vi "test - Convert config array - SGL - 1.vi"(8 "error in (no error)":errorcluster, 11 "TestCase in":refnum<class "Create New Assert Tester.lvclass">) -> (0 "error out":errorcluster, 3 "TestCase out":refnum<class "Create New Assert Tester.lvclass">)   [LabVIEW 2016, in "Create New Assert Tester.lvclass"]
uses:
  Create New Assert Tester.lvclass
  Plugins/Utility/Assert Build Configuration.ctl
  Core/Assert API Components/Failure Actions.ctl
  <vilib>/Utility/Data Type/Type Definitions/Data Type.ctl
  Plugins/Utility/Assert Scripting Configuration.ctl
  <vilib>/addons/_JKI Toolkits/VI Tester/TestCase.llb/TestCase.lvclass
  <vilib>/Utility/Data Type/NI_Data Type.lvlib
  Core/Assert API Components/Assert API Components.lvlib
  C:/Program Files (x86)/National Instruments/LabVIEW 2016/vi.lib/addons/_JKI Toolkits/VI Tester/TestCase.llb/TestCase.lvclass
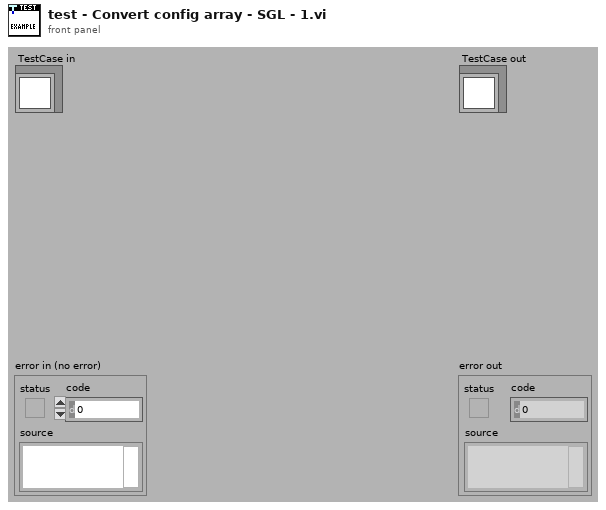
[diagram p1: front panel]
types:
  T1 = typedef "Assert Build Configuration.ctl" = cluster{"Assert Name":string, "Operation":string, "Comparison Value 1":string, "Comparison Value 2":string, "Comment":string, "Default Failure Action":T2, "Description":string, "Operation Display":string, "Active":bool, "Data Type":T3}
  T2 = typedef "Assert API Components.lvlib/Failure Actions.ctl" = enum16{"None", "Log To File", "Pause Execution", "Abort Execution"}
  T3 = typedef "NI_Data Type.lvlib/Data Type.ctl" = enum8{"Invalid Type", "Void", "I8", "I16", "I32", "I64", "U8", "U16", "U32", "U64", "Single Float", "Double Float", "Extended Float", "Single Complex", "Double Complex", "Extended Complex", "Enum U8", "Enum U16", "Enum U32", "Enum U64", "Single Float With Unit", "Double Float With Unit", "Extended Float With Unit", "Single Complex with Unit", "Double Complex with Unit", "Extended Complex with Unit", "Boolean", "String", "Path", "Picture", "Tag", "Array", "Cluster", "Variant", "LV Variant", "Waveform", "Timestamp", "Digital Waveform", "Digital Data", "ExpressData", "Refnum", "External Data", "VI", "Poly VI", "LabVIEW Class Instance", "Fixed Point"}
  T4 = enum16{"None", "Log To File", "Pause Execution", "Abort Execution"}
  T5 = typedef "Assert Scripting Configuration.ctl" = cluster{"Assert Name":string, "Comment":string, "Numeric Operation":string, "Type":T3, "String Operation":string, "DBL Comparison Value 1":dbl, "DBL Comparison Value 2":dbl, "I32 Comparison Value 1":i32, "I32 Comparison Value 2":i32, "Creator":string, "Creation Timestamp":timestamp, "String Comparison Value":string, "Description":string, "Default Failure Action":enum16{"None", "Log To File", "Pause Execution", "Abort Execution"}, "Boolean Comparison Value":bool, "I8 Comparison Value 1":i8, "I8 Comparison Value 2":i8, "I16 Comparison Value 1":i16, "I16 Comparison Value 2":i16, "I64 Comparison Value 1":i64, "I64 Comparison Value 2":i64, "U8 Comparison Value 1":u8, "U8 Comparison Value 2":u8, "U16 Comparison Value 1":u16, "U16 Comparison Value 2":u16, "U32 Comparison Value 1":u32, "U32 Comparison Value 2":u32, "U64 Comparison Value 1":u64, "U64 Comparison Value 2":u64, "EXT Comparison Value 1":ext, "EXT Comparison Value 2":ext, "SGL Comparison Value 1":sgl, "SGL Comparison Value 2":sgl}
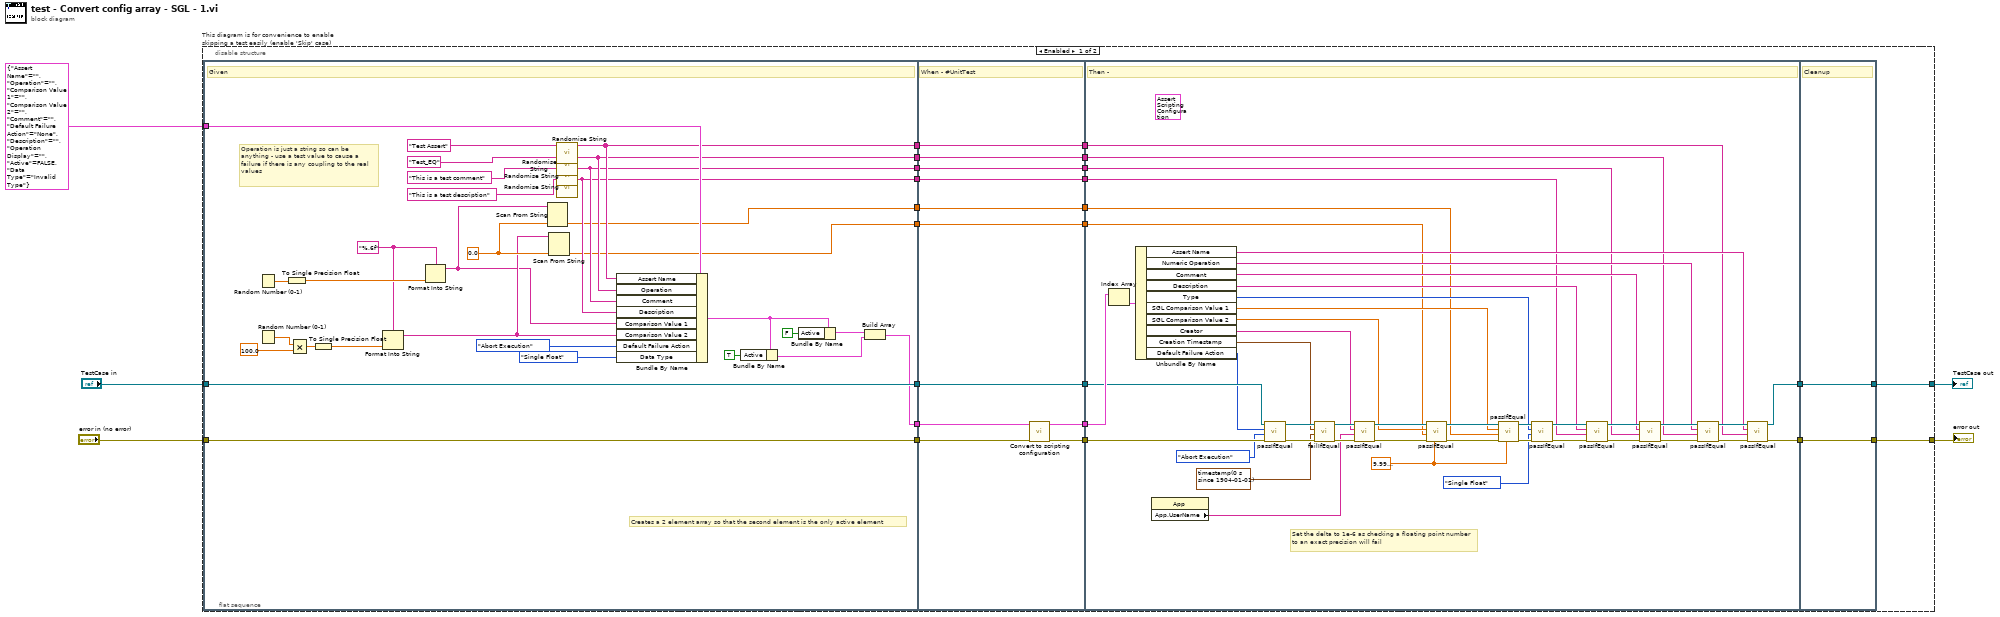
[diagram p0: block diagram]
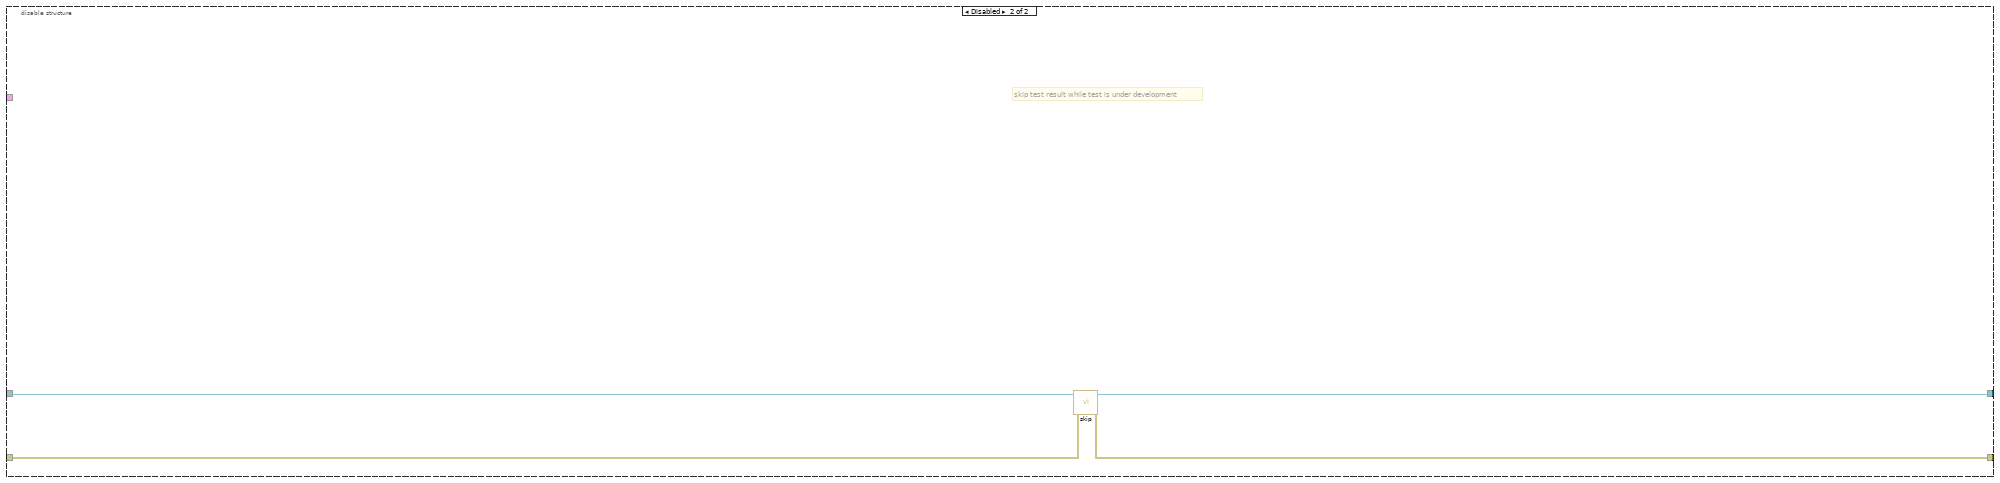
[diagram p2: hidden frame]
diagram:
  n1 = disable-structure "This diagram is for convenience to enable skipping a test easily (enable 'Skip' case)" shown="Enabled" {
    disable-tunnel: "TestCase in" -> [w24 w123]
    disable-tunnel: [w21 w121] -> w2
    disable-tunnel: [w22 w122] -> w4
    disable-tunnel: "error in (no error)" -> [w23 w120]
    disable-tunnel: T1 {"Assert Name"="", "Operation"="", "Comparison Value 1"="", "Comparison Value 2"="", "Comment"="", "Default Failure Action"=enum."None", "Description"="", "Operation Display"="", "Active"=FALSE, "Data Type"=enum."Invalid Type"} ("Assert Build Configuration") -> [w19 _]
    frame Enabled {
      n2 = flat-sequence {
        tunnel: w23 -> [w60]
        tunnel: w24 -> [w61]
        tunnel: [w61] -> w30
        tunnel: [w60] -> w29
        tunnel: w19 -> [w59]
        tunnel: [w54] -> w18
        tunnel: [w46] -> w16
        tunnel: [w45] -> w14
        tunnel: [w44] -> w12
        tunnel: [w43] -> w10
        tunnel: [w32] -> w8
        tunnel: [w31] -> w6
        tunnel: [w72] -> w28
        tunnel: [w70] -> w27
        tunnel: w30 -> [w72]
        tunnel: w29 -> [w71]
        tunnel: [w69] -> w20
        tunnel: w18 -> [w68]
        tunnel: [w67] -> w17
        tunnel: w16 -> [w67]
        tunnel: [w66] -> w15
        tunnel: w14 -> [w66]
        tunnel: [w65] -> w13
        tunnel: w12 -> [w65]
        tunnel: [w64] -> w11
        tunnel: w10 -> [w64]
        tunnel: [w63] -> w9
        tunnel: w8 -> [w63]
        tunnel: [w62] -> w7
        tunnel: w6 -> [w62]
        tunnel: [w81] -> w26
        tunnel: [w83] -> w25
        tunnel: w28 -> [w112]
        tunnel: w27 -> [w117]
        tunnel: w20 -> [w115]
        tunnel: w17 -> [w76]
        tunnel: w15 -> [w77]
        tunnel: w13 -> [w78]
        tunnel: w11 -> [w79]
        tunnel: w9 -> [w74]
        tunnel: w7 -> [w75]
        tunnel: [w118] -> w22
        tunnel: [w119] -> w21
        tunnel: w26 -> [w119]
        tunnel: w25 -> [w118]
        frame #0 {
          w35 = sgl 0.0 ("double precision float")
          w36 = "%.6f" ("format string")
          # "Creates a 2 element array so that the second element is the only active element"
          # "Operation is just a string so can be anything - use a test value to cause a failure if there is any coupling to the real values"
          # "Given"
          n3 = Random Number (0-1)() -> (number: 0 to 1=w42:dbl)
          n4 = Random Number (0-1)() -> (number: 0 to 1=w41:dbl)
          n5 = To Single Precision Float(number=w42) -> (single precision float=w37:sgl)
          n6 = Multiply(x=w41, y=100.0) -> (x*y=w39:dbl)
          n7 = To Single Precision Float(number=w39) -> (single precision float=w38:sgl)
          n8 = Format Into String(format string=w36, w38) -> (resulting string=w34:string)  [unwired: 2 in, 1 out]
          n9 = Format Into String(format string=w36, w37) -> (resulting string=w33:string)  [unwired: 2 in, 1 out]
          n10 = Scan From String(input string=w33, default 1=w35) -> (output 1=w32:sgl)  [unwired: 3 in, 3 out]
          n11 = Scan From String(input string=w34, default 1=w35) -> (output 1=w31:sgl)  [unwired: 3 in, 3 out]
          n12 = call "Randomise String.vi"("String in"="Test Assert" ("Assert Name")) -> ("String out"=w46:string)  [unwired: 10 in]
          n13 = call "Randomise String.vi"("String in"="Test_EQ" ("Operation")) -> ("String out"=w45:string)  [unwired: 10 in]
          n14 = call "Randomise String.vi"("String in"="This is a test comment" ("Comment")) -> ("String out"=w44:string)  [unwired: 10 in]
          n15 = call "Randomise String.vi"("String in"="This is a test description" ("Comment")) -> ("String out"=w43:string)  [unwired: 10 in]
          n16 = Bundle By Name(cluster=w59, "Assert Name"=w46, "Operation"=w45, "Comment"=w44, "Description"=w43, "Comparison Value 1"=w33, "Comparison Value 2"=w34, "Default Failure Action"=Failure_Actions."Abort Execution", "Data Type"=Data_Type."Single Float") -> (w51:T1)
          n17 = Bundle By Name(cluster=w51, "Active"=TRUE) -> (w49:T1)
          n18 = Bundle By Name(cluster=w51, "Active"=FALSE) -> (w53:T1)
          n19 = Build Array(w53, w49) -> (w54:T1[])
        }
        frame #1 {
          # "When - #UnitTest"
          n20 = call "Convert to scripting configuration.vi"("error in (no error)"=w71, "Multiple Assert Configuration"=w68) -> ("error out"=w70:errorcluster, "Array"=w69:T5[])  [unwired: 7 in, 1 out]
        }
        frame #2 {
          w73 = sgl 1e-06
          (unwired) T5 {"Assert Name"="", "Comment"="", "Numeric Operation"="", "Type"=enum."Invalid Type", "String Operation"="", "DBL Comparison Value 1"=0.0, "DBL Comparison Value 2"=0.0, "I32 Comparison Value 1"=0, "I32 Comparison Value 2"=0, "Creator"="", "Creation Timestamp"=timestamp(0 s since 1904-01-01), "String Comparison Value"="", "Description"="", "Default Failure Action"=enum."None", "Boolean Comparison Value"=FALSE, "I8 Comparison Value 1"=0, "I8 Comparison Value 2"=0, "I16 Comparison Value 1"=0, "I16 Comparison Value 2"=0, "I64 Comparison Value 1"=0, "I64 Comparison Value 2"=0, "U8 Comparison Value 1"=0, "U8 Comparison Value 2"=0, "U16 Comparison Value 1"=0, "U16 Comparison Value 2"=0, "U32 Comparison Value 1"=0, "U32 Comparison Value 2"=0, "U64 Comparison Value 1"=0, "U64 Comparison Value 2"=0, "EXT Comparison Value 1"=0.0, "EXT Comparison Value 2"=0.0, "SGL Comparison Value 1"=0.0, "SGL Comparison Value 2"=0.0} ("Assert Scripting Configuration")
          # "Set the delta to 1e-6 as checking a floating point number to an exact precision will fail"
          # "Then -"
          n21 = Index Array(array=w115) -> (element=w114:T5)  [unwired: 1 in]
          n22 = Unbundle By Name(w114) -> ("Assert Name"=w80:string, "Numeric Operation"=w89:string, "Comment"=w90:string, "Description"=w91:string, "Type"=w92:T3, "SGL Comparison Value 1"=w99:sgl, "SGL Comparison Value 2"=w100:sgl, "Creator"=w101:string, "Creation Timestamp"=w87:timestamp, "Default Failure Action"=w110:T4)
          n23 = property class="App"() -> ("App.UserName"=w85:string)  [unwired: 2 in, 2 out]
          n24 = call-dynamic "passIfEqual.vi"("error in (no error)"=w117, "y"=T4."Abort Execution" ("Default Failure Action"), "x"=w110, "TestCase in"=w112) -> ("error out"=w113:errorcluster, "TestCase out"=w111:refnum<class "Create New Assert Tester.lvclass">)  [unwired: 6 in]
          n25 = call-dynamic "failIfEqual.vi"("error in (no error)"=w113, "y"=timestamp(0 s since 1904-01-01) ("Creation Timestamp"), "x"=w87, "TestCase in"=w111) -> ("error out"=w116:errorcluster, "TestCase out"=w106:refnum<class "Create New Assert Tester.lvclass">)  [unwired: 6 in]
          n26 = call-dynamic "passIfEqual.vi"("error in (no error)"=w116, "y"=w85, "x"=w101, "TestCase in"=w106) -> ("error out"=w107:errorcluster, "TestCase out"=w105:refnum<class "Create New Assert Tester.lvclass">)  [unwired: 6 in]
          n27 = call-dynamic "passIfEqual.vi"("delta (optional)"=w73, "error in (no error)"=w107, "y"=w75, "x"=w100, "TestCase in"=w105) -> ("error out"=w108:errorcluster, "TestCase out"=w103:refnum<class "Create New Assert Tester.lvclass">)  [unwired: 5 in]
          n28 = call-dynamic "passIfEqual.vi"("delta (optional)"=w73, "error in (no error)"=w108, "y"=w74, "x"=w99, "TestCase in"=w103) -> ("error out"=w104:errorcluster, "TestCase out"=w97:refnum<class "Create New Assert Tester.lvclass">)  [unwired: 5 in]
          n29 = call-dynamic "passIfEqual.vi"("error in (no error)"=w104, "y"=Data_Type."Single Float" ("Data Type"), "x"=w92, "TestCase in"=w97) -> ("error out"=w98:errorcluster, "TestCase out"=w96:refnum<class "Create New Assert Tester.lvclass">)  [unwired: 6 in]
          n30 = call-dynamic "passIfEqual.vi"("error in (no error)"=w98, "y"=w79, "x"=w91, "TestCase in"=w96) -> ("error out"=w102:errorcluster, "TestCase out"=w94:refnum<class "Create New Assert Tester.lvclass">)  [unwired: 6 in]
          n31 = call-dynamic "passIfEqual.vi"("error in (no error)"=w102, "y"=w78, "x"=w90, "TestCase in"=w94) -> ("error out"=w95:errorcluster, "TestCase out"=w93:refnum<class "Create New Assert Tester.lvclass">)  [unwired: 6 in]
          n32 = call-dynamic "passIfEqual.vi"("error in (no error)"=w95, "y"=w77, "x"=w89, "TestCase in"=w93) -> ("error out"=w109:errorcluster, "TestCase out"=w82:refnum<class "Create New Assert Tester.lvclass">)  [unwired: 6 in]
          n33 = call-dynamic "passIfEqual.vi"("error in (no error)"=w109, "y"=w76, "x"=w80, "TestCase in"=w82) -> ("error out"=w83:errorcluster, "TestCase out"=w81:refnum<class "Create New Assert Tester.lvclass">)  [unwired: 6 in]
        }
        frame #3 {
          # "Cleanup"
        }
      }
    }
    frame Disabled {
      # "skip test result while test is under development"
      n34 = call <vilib>:"skip.vi"("error in (no error)"=w120, "TestCase in"=w123) -> ("error out"=w122:errorcluster, "TestCase out"=w121:refnum<class "Create New Assert Tester.lvclass">)  [unwired: 8 in]
    }
  }
  "error out" <- w4
  "TestCase out" <- w2
